vi "Configure Trigger Characteristics (TV).vi"(5 "Line Number (17)":i32=17, 6 "Enable TV Monitor (T: Enable)":bool=TRUE, 7 "TV Field (0: Entire)":u16(ring) items=["Entire", "Field 1", "Field 2"], 8 "error in (no error)":errorcluster, 9 "TV Signal Format (0: NTSC-M)":u16(ring) items=["NTSC-M", "NTSC-Japan", "PAL-M", "PAL-B,D,G,H,I", "PAL-N", "PAL-N Combin", "SECAM-L"], 10 "TV Source (0: Spectrum Analyzer)":u16(ring) items=["Spectrum Analyzer", "External"], 11 "VISA resource name":refnum<visa-resource-name>) -> (0 "error out":errorcluster, 3 "VISA resource name out":refnum<visa-resource-name>)   [LabVIEW 2014, in "Agilent ESA PSA Series.lvlib"]
doc: "Configures the trigger settings for TV trigger on the spectrum analyzer.It is applicable when the trigger source is set to TV trigger and Options BAA and B7B are installed."
uses:
  Agilent ESA PSA Series.lvlib
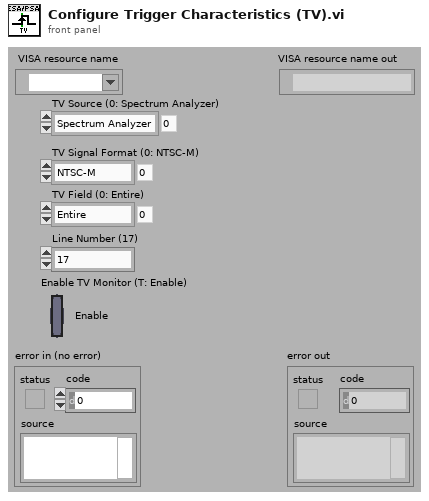
[diagram p1: front panel]
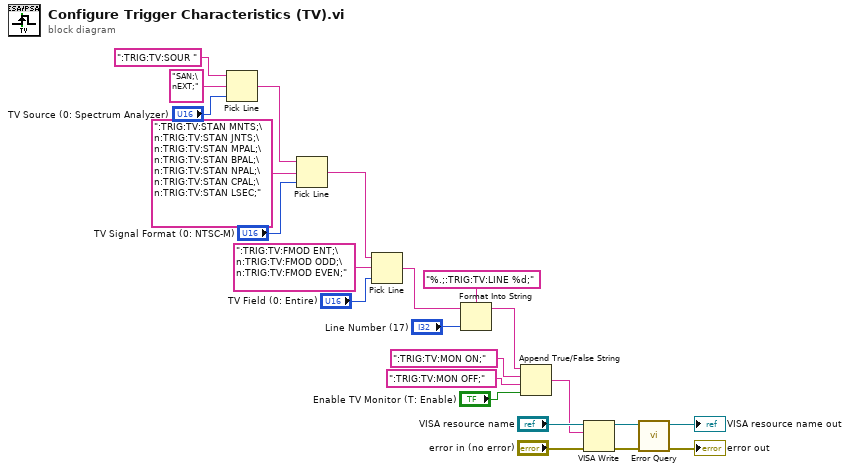
[diagram p0: block diagram]
diagram:
  n1 = Pick Line(string ("")=":TRIG:TV:SOUR ", multi-line string="SAN;\nEXT;", line index="TV Source (0: Spectrum Analyzer)") -> (output string=w11:string)
  n2 = Pick Line(string ("")=w11, multi-line string=":TRIG:TV:STAN MNTS;\n:TRIG:TV:STAN JNTS;\n:TRIG:TV:STAN MPAL;\n:TRIG:TV:STAN BPAL;\n:TRIG:TV:STAN NPAL;\n:TRIG:TV:STAN CPAL;\n:TRIG:TV:STAN LSEC;", line index="TV Signal Format (0: NTSC-M)") -> (output string=w6:string)
  n3 = Pick Line(string ("")=w6, multi-line string=":TRIG:TV:FMOD ENT;\n:TRIG:TV:FMOD ODD;\n:TRIG:TV:FMOD EVEN;", line index="TV Field (0: Entire)") -> (output string=w4:string)
  n4 = Format Into String(format string="%.;:TRIG:TV:LINE %d;", initial string=w4, "Line Number (17)") -> (resulting string=w2:string)  [unwired: 1 in, 1 out]
  n5 = Append True/False String(1:"Enable TV Monitor (T: Enable)", 2:":TRIG:TV:MON OFF;" ("true string"), 3:":TRIG:TV:MON ON;" ("true string"), 4:w2) -> (0:w1:string)
  n6 = VISA Write(VISA resource name="VISA resource name", write buffer=w1, error in (no error)="error in (no error)") -> (VISA resource name out=w21:refnum<visa-resource-name>, error out=w19:errorcluster)  [unwired: 1 out]
  n7 = call "Error Query.vi"("error in (no error)"=w19, "VISA resource name"=w21) -> ("error out"=→"error out":errorcluster, "VISA resource name out"=→"VISA resource name out":refnum<visa-resource-name>)  [unwired: 6 in, 2 out]
